vi "Save_current_command.vi"(2 "Array":u8[](array[numeric])) -> ()   [LabVIEW 2016]
uses:
  Global_Valves.vi
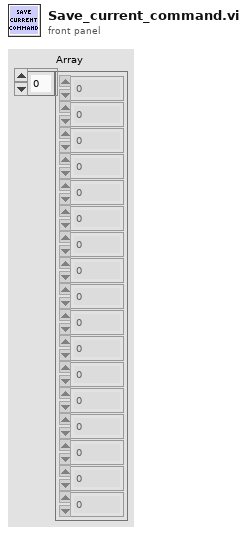
[diagram p1: front panel]
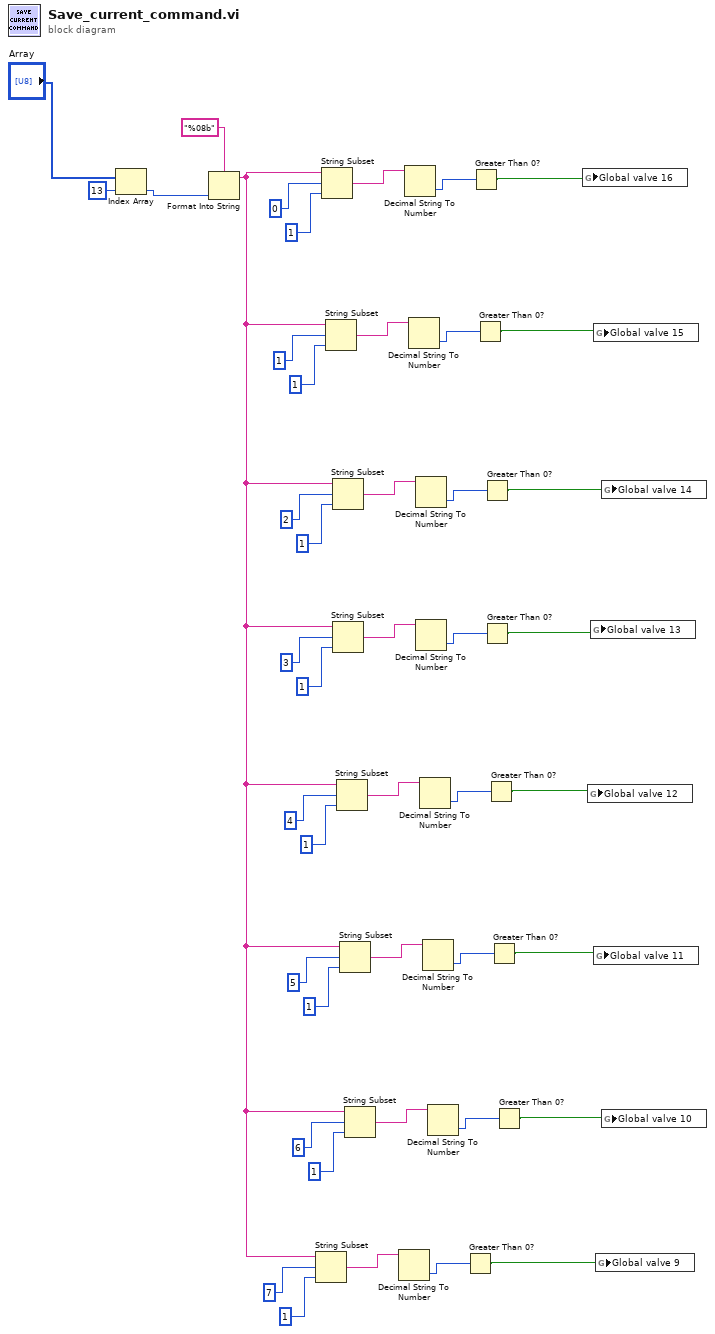
[diagram p0: block diagram]
diagram:
  n1 = Index Array(array="Array", index=13) -> (element=w3:u8)
  n2 = Format Into String(format string="%08b", w3) -> (resulting string=w1:string)  [unwired: 2 in, 1 out]
  n3 = String Subset(string=w1, offset (0)=7, length (rest)=1 ("length (rest)")) -> (substring=w43:string)
  n4 = String Subset(string=w1, offset (0)=0, length (rest)=1 ("length (rest)")) -> (substring=w16:string)
  n5 = String Subset(string=w1, offset (0)=1, length (rest)=1 ("length (rest)")) -> (substring=w19:string)
  n6 = String Subset(string=w1, offset (0)=2, length (rest)=1 ("length (rest)")) -> (substring=w24:string)
  n7 = String Subset(string=w1, offset (0)=3, length (rest)=1 ("length (rest)")) -> (substring=w27:string)
  n8 = String Subset(string=w1, offset (0)=4, length (rest)=1 ("length (rest)")) -> (substring=w32:string)
  n9 = String Subset(string=w1, offset (0)=5, length (rest)=1 ("length (rest)")) -> (substring=w35:string)
  n10 = String Subset(string=w1, offset (0)=6, length (rest)=1 ("length (rest)")) -> (substring=w40:string)
  n11 = Decimal String To Number(string=w43) -> (number=w42:i32)  [unwired: 2 in, 1 out]
  n12 = Decimal String To Number(string=w16) -> (number=w17:i32)  [unwired: 2 in, 1 out]
  n13 = Decimal String To Number(string=w19) -> (number=w18:i32)  [unwired: 2 in, 1 out]
  n14 = Decimal String To Number(string=w24) -> (number=w25:i32)  [unwired: 2 in, 1 out]
  n15 = Decimal String To Number(string=w27) -> (number=w26:i32)  [unwired: 2 in, 1 out]
  n16 = Decimal String To Number(string=w32) -> (number=w33:i32)  [unwired: 2 in, 1 out]
  n17 = Decimal String To Number(string=w35) -> (number=w34:i32)  [unwired: 2 in, 1 out]
  n18 = Decimal String To Number(string=w40) -> (number=w41:i32)  [unwired: 2 in, 1 out]
  n19 = Greater Than 0?(x=w42) -> (x > 0?=w4:bool)
  n20 = Greater Than 0?(x=w17) -> (x > 0?=w11:bool)
  n21 = Greater Than 0?(x=w18) -> (x > 0?=w10:bool)
  n22 = Greater Than 0?(x=w25) -> (x > 0?=w9:bool)
  n23 = Greater Than 0?(x=w26) -> (x > 0?=w8:bool)
  n24 = Greater Than 0?(x=w33) -> (x > 0?=w7:bool)
  n25 = Greater Than 0?(x=w34) -> (x > 0?=w6:bool)
  n26 = Greater Than 0?(x=w41) -> (x > 0?=w5:bool)
  n27 = global write "Global_Valves.vi" "Global valve 16"(w11) -> ()
  n28 = global write "Global_Valves.vi" "Global valve 12"(w7) -> ()
  n29 = global write "Global_Valves.vi" "Global valve 13"(w8) -> ()
  n30 = global write "Global_Valves.vi" "Global valve 15"(w10) -> ()
  n31 = global write "Global_Valves.vi" "Global valve 11"(w6) -> ()
  n32 = global write "Global_Valves.vi" "Global valve 9"(w4) -> ()
  n33 = global write "Global_Valves.vi" "Global valve 14"(w9) -> ()
  n34 = global write "Global_Valves.vi" "Global valve 10"(w5) -> ()
